vi "globals2.vi"() -> ()   [LabVIEW 2011]
panel:
  in  "Quad D/A Card 5 Slot":u16(ring)=9 items=["400@", "401A", "402B", "403C", "404D", "405E", "406F", "407G", "408H", "409I", "410J", "411K", "412L", "413M", "414N"]
  in  "Quad D/A Card 4 Slot":u16(ring)=8 items=["400@", "401A", "402B", "403C", "404D", "405E", "406F", "407G", "408H", "409I", "410J", "411K", "412L", "413M", "414N"]
  in  "Quad D/A Card 3 Slot":u16(ring)=7 items=["400@", "401A", "402B", "403C", "404D", "405E", "406F", "407G", "408H", "409I", "410J", "411K", "412L", "413M", "414N"]
  in  "Quad D/A Card 2 Slot":u16(ring)=5 items=["400@", "401A", "402B", "403C", "404D", "405E", "406F", "407G", "408H", "409I", "410J", "411K", "412L", "413M", "414N"]
  in  "Quad D/A Card 1 Slot":u16(ring)=4 items=["400@", "401A", "402B", "403C", "404D", "405E", "406F", "407G", "408H", "409I", "410J", "411K", "412L", "413M", "414N"]
  in  "Relay Card 5 Slot":u16(ring)=14 items=["400@", "401A", "402B", "403C", "404D", "405E", "406F", "407G", "408H", "409I", "410J", "411K", "412L", "413M", "414N"]
  in  "Relay Card 4 Slot":u16(ring)=13 items=["400@", "401A", "402B", "403C", "404D", "405E", "406F", "407G", "408H", "409I", "410J", "411K", "412L", "413M", "414N"]
  in  "Relay Card 3 Slot":u16(ring)=12 items=["400@", "401A", "402B", "403C", "404D", "405E", "406F", "407G", "408H", "409I", "410J", "411K", "412L", "413M", "414N"]
  in  "Relay Card 2 Slot":u16(ring)=11 items=["400@", "401A", "402B", "403C", "404D", "405E", "406F", "407G", "408H", "409I", "410J", "411K", "412L", "413M", "414N"]
  in  "Relay Card 1 Slot":u16(ring)=10 items=["400@", "401A", "402B", "403C", "404D", "405E", "406F", "407G", "408H", "409I", "410J", "411K", "412L", "413M", "414N"]
  in  "Timer Slot":u16(ring)=2 items=["400@", "401A", "402B", "403C", "404D", "405E", "406F", "407G", "408H", "409I", "410J", "411K", "412L", "413M", "414N"]
  in  "High-Speed A/D Slot":u16(ring)=1 items=["400@", "401A", "402B", "403C", "404D", "405E", "406F", "407G", "408H", "409I", "410J", "411K", "412L", "413M", "414N"]
  in  "Scanner Slot":u16(ring) items=["400@", "401A", "402B", "403C", "404D", "405E", "406F", "407G", "408H", "409I", "410J", "411K", "412L", "413M", "414N"]
  out "Growth Sequence Preferences":path=path "C:/MOCVD/GrowthSequencePreferences.ini"
  out "Growth Database":path=path "C:/MOCVD/MOCVD_Growths.accdb"
  out "Log Path":path
  out "Last Step":i32
  out "Seq Step Time (s)":dbl=0.01
  out "Current Time":timestamp
  out "Begin Time":timestamp
  out "Temperature Controller RS232":refnum<visa-resource-name>="COM1"
  out "Log String":string
  out "Byte Stream File Refnum":refnum<file>
  out "Log File Path":path
  out "GPIB Address":string="23"
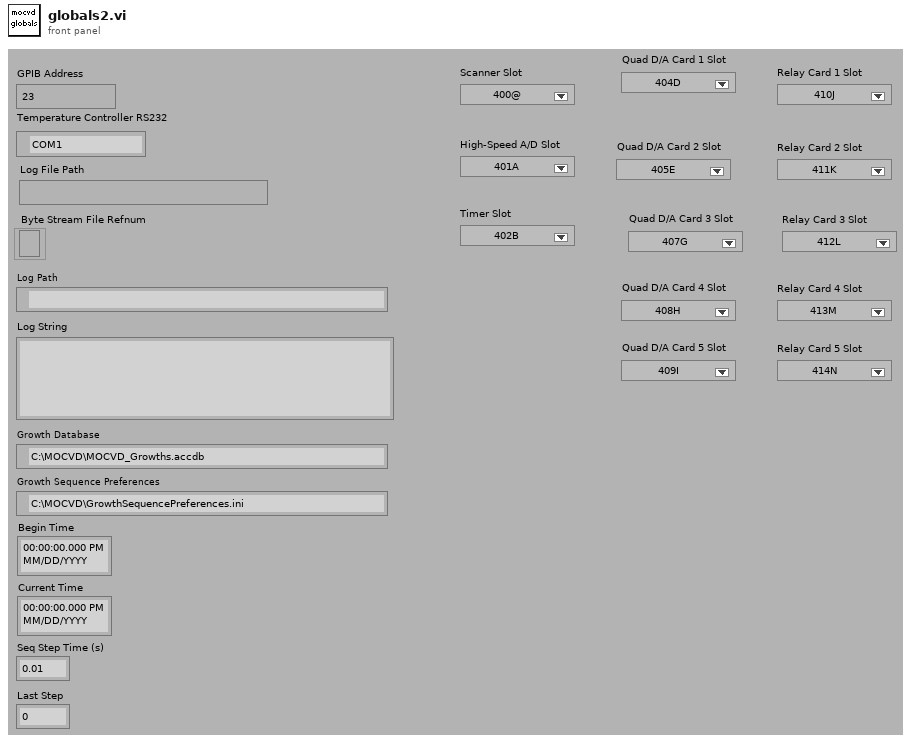
[diagram p1: front panel]
diagram:
